vi "Write Return Device Generation Mode Msg.vi"(10 "Return Device Generation Mode Msg":refnum<class "Return Device Generation Mode Msg.lvclass">, 11 "Optimization in":refnum<class "Optimization.lvclass">) -> (3 "Optimization out":refnum<class "Optimization.lvclass">)   [LabVIEW 2016, in "Optimization Framework.lvlib" / "Optimization.lvclass"]
uses:
  Optimization.lvclass
  Optimization Messages/Return Device Generation Mode Msg/Return Device Generation Mode Msg.lvclass
  Optimization.lvclass/Optimization.ctl
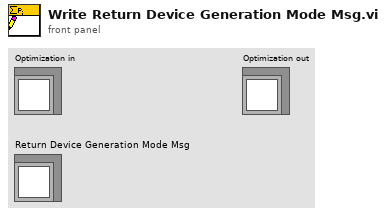
[diagram p1: front panel]
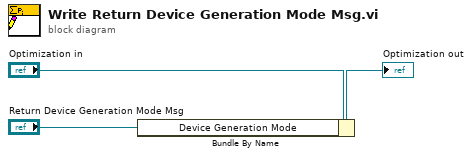
[diagram p0: block diagram]
diagram:
  n1 = Bundle By Name(cluster="Optimization in", "Device Generation Mode"="Return Device Generation Mode Msg") -> (→"Optimization out":refnum<class "Optimization.lvclass">)
